vi "Read Phases.vi"(8 "error in (no error)":errorcluster, 11 "Lockin Digitizer Driver in":refnum<class "Lockin Digitizer Driver.lvclass">) -> (0 "error out":errorcluster, 2 "Phases":dbl[](array[numeric]), 3 "Lockin Digitizer Driver out":refnum<class "Lockin Digitizer Driver.lvclass">)   [LabVIEW 2024, in "Lockin Digitizer Driver.lvclass"]
uses:
  Lockin Digitizer Driver.lvclass
  Lockin Digitizer Driver.lvclass/Lockin Digitizer Driver.ctl
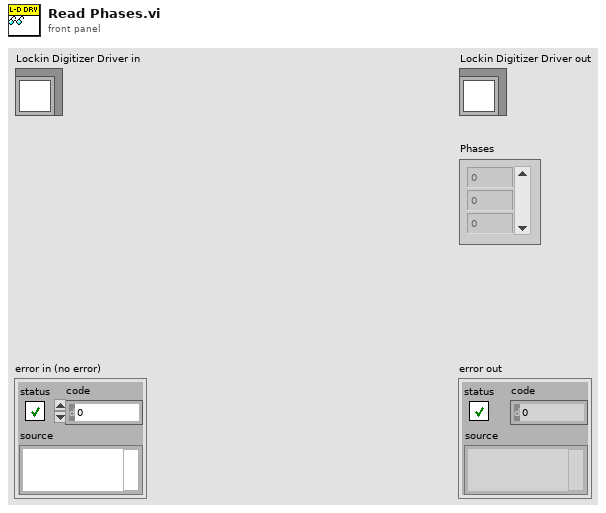
[diagram p1: front panel]
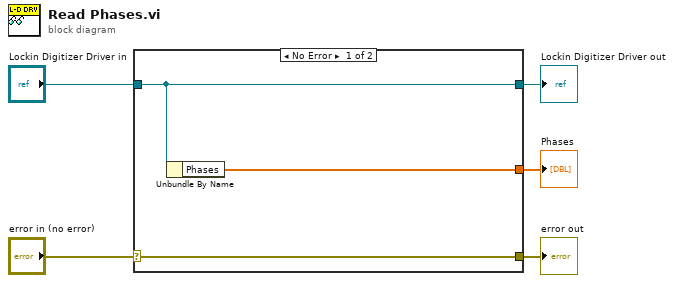
[diagram p0: block diagram]
diagram:
  n1 = case shown="No Error" "error in (no error)" {
    selector: "error in (no error)" -> [w8 w9]
    tunnel: [w8 w9] -> w4
    tunnel: [w7 w10] -> w2
    tunnel: "Lockin Digitizer Driver in" -> [w7 w10]
    tunnel: [w6 _] -> w1
    frame No Error {
      n2 = Unbundle By Name(w7) -> ("Phases"=w6:dbl[])
    }
    frame Error {
    }
  }
  "error out" <- w4
  "Lockin Digitizer Driver out" <- w2
  "Phases" <- w1
